vi "Test_FormatNames_CommonTypes_NamesOK.vi"(8 "error in (no error)":errorcluster, 11 "TestCase in":refnum<class "TestVariantExtensions.lvclass">) -> (0 "error out":errorcluster, 3 "TestCase out":refnum<class "TestVariantExtensions.lvclass">)   [LabVIEW 2017, in "TestVariantExtensions.lvclass"]
uses:
  TestVariantExtensions.lvclass
  Source/VariantExtensions.lvlib
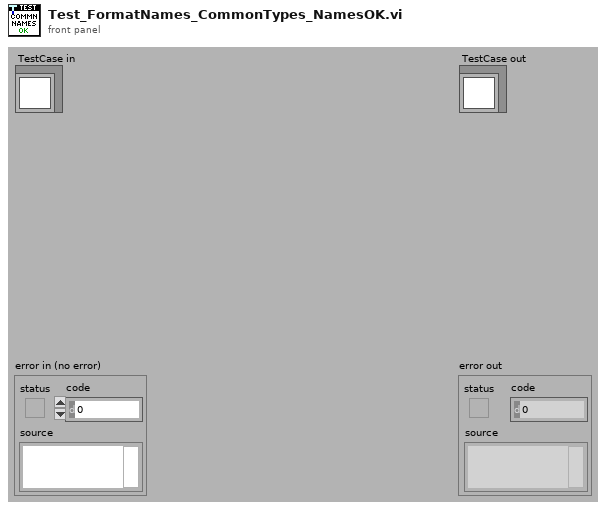
[diagram p1: front panel]
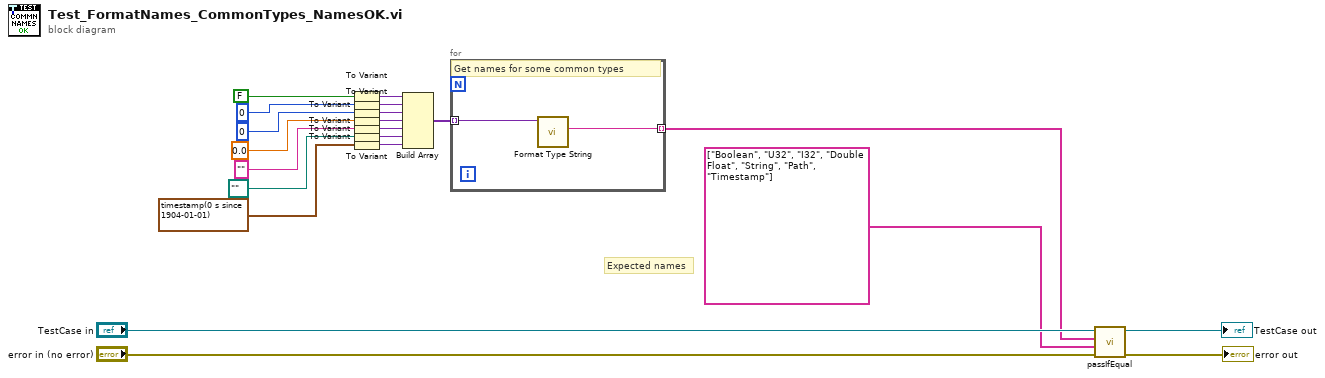
[diagram p0: block diagram]
diagram:
  # "Expected names"
  n1 = To Variant(anything=FALSE) -> (Variant=w1:variant)
  n2 = To Variant(anything=u32 0) -> (Variant=w17:variant)
  n3 = To Variant(anything=0) -> (Variant=w16:variant)
  n4 = To Variant(anything=0.0) -> (Variant=w15:variant)
  n5 = To Variant(anything="") -> (Variant=w14:variant)
  n6 = To Variant(anything=path "") -> (Variant=w13:variant)
  n7 = To Variant(anything=timestamp(0 s since 1904-01-01)) -> (Variant=w12:variant)
  n8 = Build Array(w1, w17, w16, w15, w14, w13, w12) -> (w5:variant[])
  n9 = for {
    tunnel: [w23] -> w4 mode=indexing
    tunnel: w5 -> [w22] mode=indexing
    # "Get names for some common types"
    n10 = call "Format Type String.vi"("Data Type"=w22) -> ("Type Name"=w23:string)  [unwired: 9 in, 1 out]
  }
  n11 = call-dynamic "passIfEqual.vi"("error in (no error)"="error in (no error)", "y"=string[] ["Boolean", "U32", "I32", "Double Float", "String", "Path", "Timestamp"], "x"=w4, "TestCase in"="TestCase in") -> ("error out"=→"error out":errorcluster, "TestCase out"=→"TestCase out":refnum<class "TestVariantExtensions.lvclass">)  [unwired: 6 in]
